vi "HW_Poll_Tracker_2.0.3.vi"(8 "error in":errorcluster, 11 "VISA resource name in":refnum<visa-resource-name>="ASRL3::INSTR") -> (0 "error out":errorcluster, 1 "Read buffer":string, 2 "Parameters output":T1, 3 "VISA resource name out":refnum<visa-resource-name>, 5 "Sensor board size":string)   [LabVIEW 2018, in "HW Interaction.lvlib"]
uses:
  HW Interaction.lvlib
  <vilib>/Utility/error.llb/Error Cluster From Error Code.vi
  <vilib>/ErrorRing/Error Ring.xnode
panel:
  out "Sensors response":string
  out "Port data status":i32
  out "Port data status index":i32
  out "FPS status":i32
  out "Poll records":u32
  out "FPS target index":i32
  out "Matrix mode status":string
  out "Matrix mode index":i32
  out "Coordinate mode status":string
  out "Coordinate mode index":i32
  out "Binary mode status":string
  out "Binary mode index":i32
  out "Array of tokens":string[](array[string])
  out "token index":i32
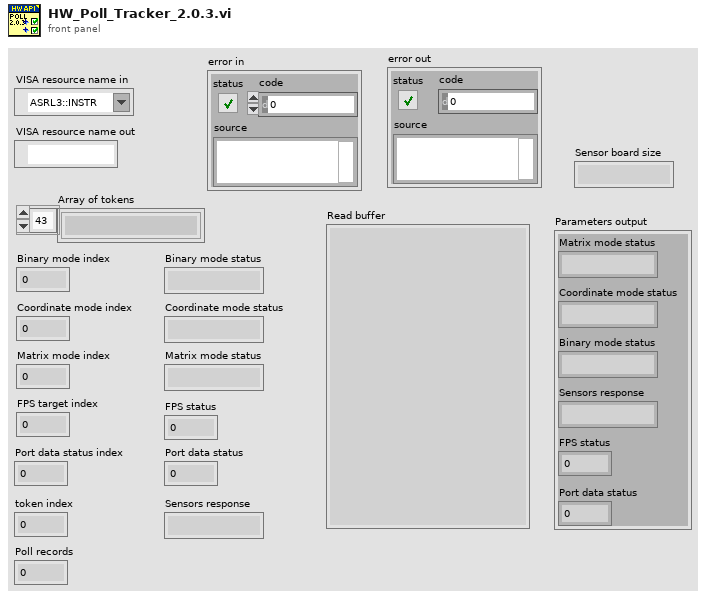
[diagram p1: front panel]
types:
  T1 = cluster{"Matrix mode status":string, "Coordinate mode status":string, "Binary mode status":string, "Sensors response":string, "FPS status":i32, "Port data status":i32}
  T2 = cluster{"token string":string, "token string":string, "token string":string, "trimmed string":string, i32, i32}
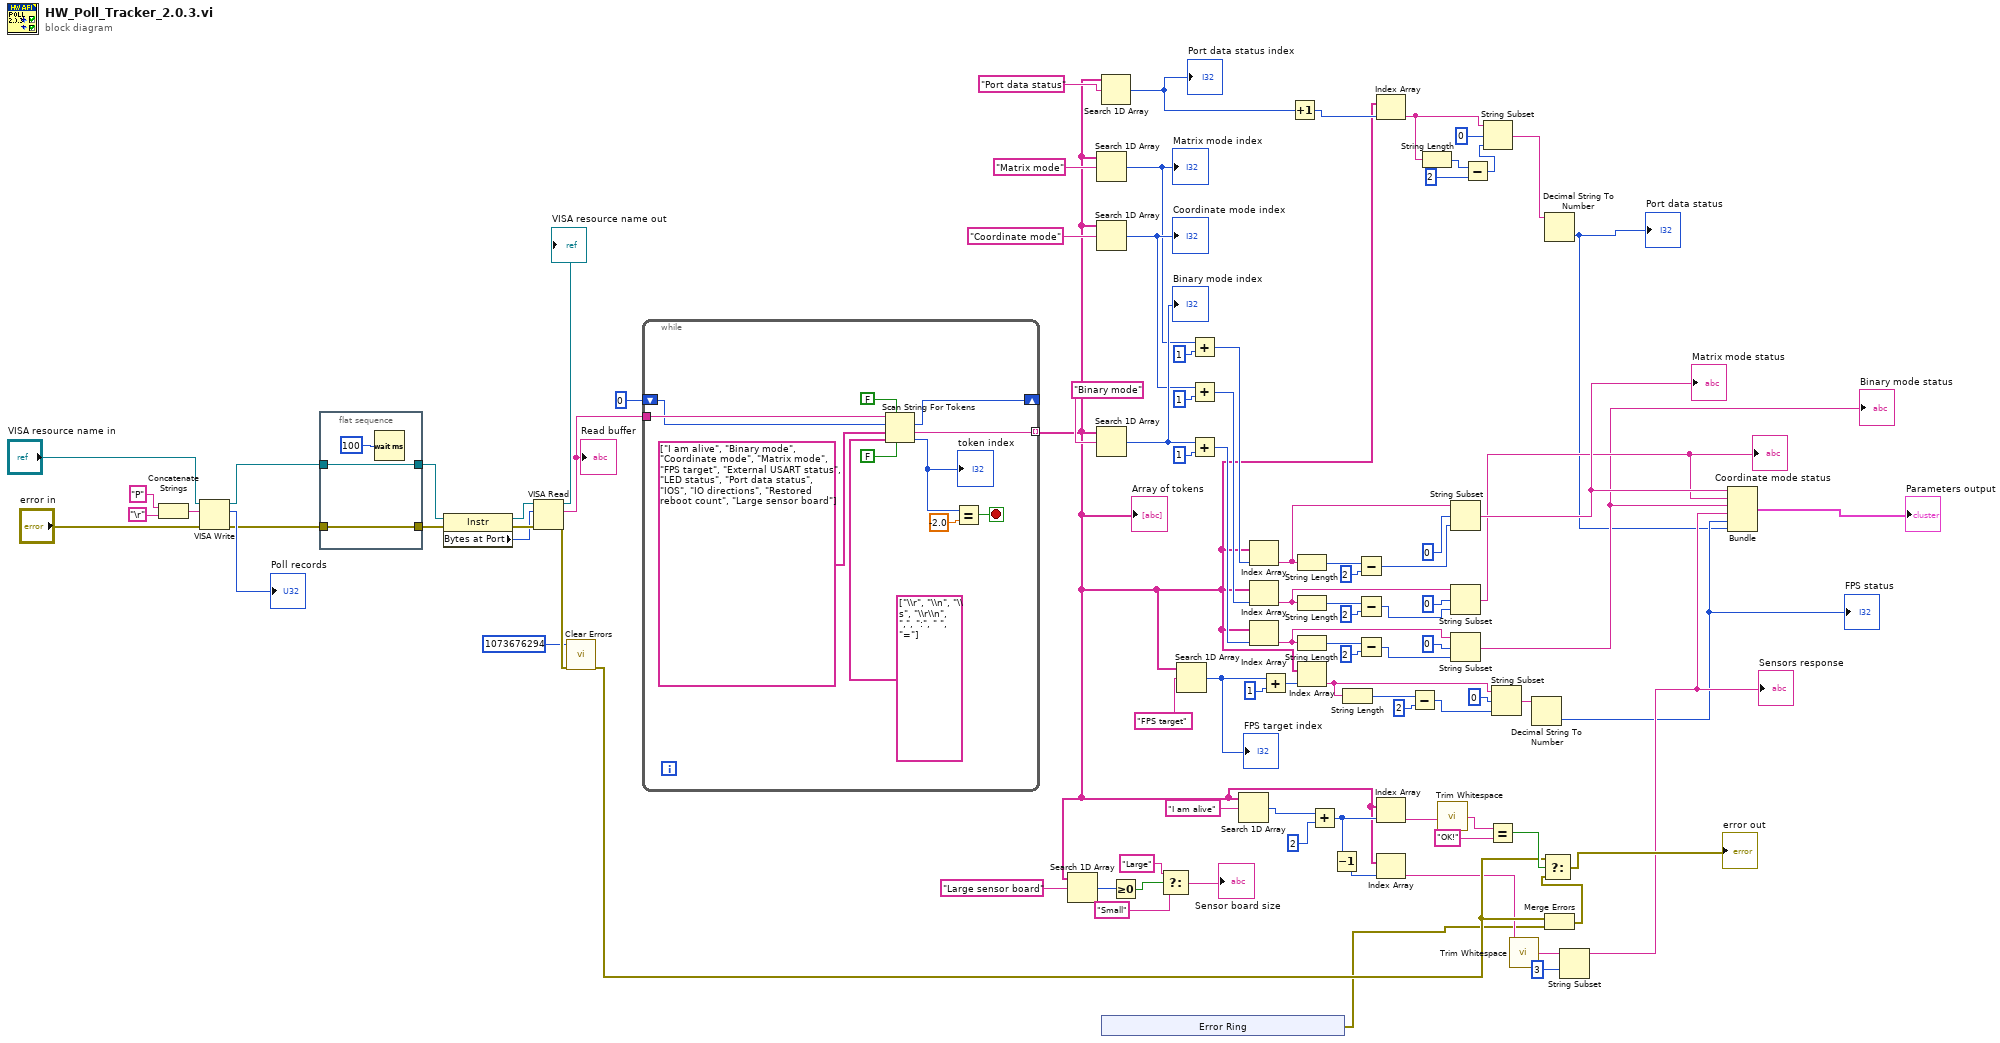
[diagram p0: block diagram]
diagram:
  n1 = Concatenate Strings("P" ("write buffer"), "\r") -> (w92:string)
  n2 = VISA Write(VISA resource name="VISA resource name in", write buffer=w92, error in (no error)="error in") -> (VISA resource name out=w67:refnum<visa-resource-name>, return count=→"Poll records":u32, error out=w65:errorcluster)
  n3 = flat-sequence {
    tunnel: [w96] -> w68
    tunnel: w67 -> [w96]
    tunnel: [w95] -> w66
    tunnel: w65 -> [w95]
    frame #0 {
      n4 = Wait (ms)(milliseconds to wait=u32 100) -> ()  [unwired: 1 out]
    }
  }
  n5 = property class="Instr"(reference=w68, error in=w66) -> (reference out=w90:refnum<visa-resource-name>, error out=w89:errorcluster, "Bytes at Port"=w88:u32)
  n6 = VISA Read(VISA resource name=w90, byte count=w88, error in (no error)=w89) -> (VISA resource name out=→"VISA resource name out":refnum<visa-resource-name>, read buffer=w87:string, error out=w24:errorcluster)  [unwired: 1 out]
  "Read buffer" <- w87
  n7 = call <vilib>:"Clear Errors.vi"("error in (no error)"=w24, "specific error code to clear (0: all)"=1073676294) -> ("error out"=w23:errorcluster)  [unwired: 4 in, 1 out]
  n8 = while {
    tunnel: w87 -> [w108]
    tunnel: [w100] -> w9 mode=indexing
    shift-right: [w99] -> _
    shift-left: 0 ("offset past token") -> [w98]
    stop <- w106 stop-if-true
    n9 = Scan String For Tokens(4:FALSE ("use cached delim/oper data? (F)"), 5:FALSE ("allow empty tokens? (F)"), 6:string[] ["\\r", "\\n", "\\s", "\\r\\n", ",", ":", " ", "="] ("delimiters"), 7:string[] ["I am alive", "Binary mode", "Coordinate mode", "Matrix mode", "FPS target", "External USART status", "LED status", "Port data status", "IOS", "IO directions", "Restored reboot count", "Large sensor board"] ("Tokens"), 8:w98, 9:w108) -> (0:w104:i32, 1:w100:string, 2:w99:i32)  [unwired: 1 out]
    "token index" <- w104
    n10 = Equal?(x=w104, y=-2.0) -> (x = y?=w106:bool)
  }
  "Array of tokens" <- w9
  n11 = Search 1D Array(1D array=w9, element="Large sensor board") -> (index of element=w7:i32)  [unwired: 1 in]
  n12 = Search 1D Array(1D array=w9, element="Matrix mode") -> (index of element=w76:i32)  [unwired: 1 in]
  "Matrix mode index" <- w76
  n13 = Search 1D Array(1D array=w9, element="Coordinate mode") -> (index of element=w80:i32)  [unwired: 1 in]
  "Coordinate mode index" <- w80
  n14 = Search 1D Array(1D array=w9, element="Binary mode") -> (index of element=w84:i32)  [unwired: 1 in]
  "Binary mode index" <- w84
  n15 = Search 1D Array(1D array=w9, element="Port data status") -> (index of element=w41:i32)  [unwired: 1 in]
  "Port data status index" <- w41
  n16 = xnode "Error Ring"() -> ("error out"=w1:errorcluster)
  n17 = Greater Or Equal To 0?(x=w7) -> (x >= 0?=w6:bool)
  n18 = Select(t="Large", s=w6, f="Small") -> (s? t:f=→"Sensor board size":string)
  n19 = Search 1D Array(1D array=w9, element="FPS target") -> (index of element=w72:i32)  [unwired: 1 in]
  "FPS target index" <- w72
  n20 = Add(x=w76, y=1) -> (x+y=w77:i32)
  n21 = Add(x=w80, y=1) -> (x+y=w81:i32)
  n22 = Add(x=w84, y=1) -> (x+y=w85:i32)
  n23 = Search 1D Array(1D array=w9, element="I am alive") -> (index of element=w32:i32)  [unwired: 1 in]
  n24 = Index Array(array=w9, index=w77) -> (element=w45:string)
  n25 = Index Array(array=w9, index=w81) -> (element=w43:string)
  n26 = Index Array(array=w9, index=w85) -> (element=w62:string)
  n27 = Add(x=w72, y=1) -> (x+y=w73:i32)
  n28 = Increment(x=w41) -> (x+1=w40:i32)
  n29 = String Length(string=w45) -> (length=w57:i32)
  n30 = String Length(string=w43) -> (length=w48:i32)
  n31 = String Length(string=w62) -> (length=w61:i32)
  n32 = Index Array(array=w9, index=w73) -> (element=w44:string)
  n33 = Add(x=w32, y=2) -> (x+y=w21:i32)
  n34 = Decrement(x=w21) -> (x-1=w20:i32)
  n35 = String Length(string=w44) -> (length=w53:i32)
  n36 = Subtract(x=w57, y=2) -> (x-y=w55:i32)
  n37 = Subtract(x=w48, y=2) -> (x-y=w46:i32)
  n38 = Subtract(x=w61, y=2) -> (x-y=w59:i32)
  n39 = Index Array(array=w9, index=w40) -> (element=w39:string)
  n40 = Index Array(array=w9, index=w21) -> (element=w30:string)
  n41 = Index Array(array=w9, index=w20) -> (element=w19:string)
  n42 = Subtract(x=w53, y=2) -> (x-y=w51:i32)
  n43 = String Length(string=w39) -> (length=w38:i32)
  n44 = call <vilib>:"Trim Whitespace.vi"("string"=w30) -> ("trimmed string"=w29:string)  [unwired: 1 in]
  n45 = String Subset(string=w45, offset (0)=0, length (rest)=w55) -> (substring=w16:string)
  "Matrix mode status" <- w16
  n46 = String Subset(string=w43, offset (0)=0, length (rest)=w46) -> (substring=w15:string)
  "Coordinate mode status" <- w15
  n47 = String Subset(string=w62, offset (0)=0, length (rest)=w59) -> (substring=w14:string)
  "Binary mode status" <- w14
  n48 = Subtract(x=w38, y=2) -> (x-y=w36:i32)
  n49 = String Subset(string=w39, offset (0)=0, length (rest)=w36) -> (substring=w34:string)
  n50 = Equal?(x=w29, y="OK!") -> (x = y?=w27:bool)
  n51 = String Subset(string=w44, offset (0)=0, length (rest)=w51) -> (substring=w50:string)
  n52 = call <vilib>:"Trim Whitespace.vi"("string"=w19) -> ("trimmed string"=w18:string)  [unwired: 1 in]
  n53 = Decimal String To Number(string=w50) -> (number=w12:i32)  [unwired: 2 in, 1 out]
  "FPS status" <- w12
  n54 = Decimal String To Number(string=w34) -> (number=w11:i32)  [unwired: 2 in, 1 out]
  "Port data status" <- w11
  n55 = Merge Errors(w23, w1) -> (w25:errorcluster)
  n56 = Select(t=w23, s=w27, f=w25) -> (s? t:f=→"error out":errorcluster)
  n57 = String Subset(string=w18, offset (0)=3) -> (substring=w13:string)  [unwired: 1 in]
  "Sensors response" <- w13
  n58 = Bundle("token string"=w16, "token string"=w15, "token string"=w14, "trimmed string"=w13, w12, w11) -> (→"Parameters output":T2)  [unwired: 1 in]
